vi "Generate INL Straight Lines.vi"(0 "Actual voltage array":dbl[](array[numeric]), 5 "INL Method":T1, 11 "Error In":errorcluster) -> (4 "Straight Line":dbl[](graph), 15 "Error Out":errorcluster)   [LabVIEW 2023]
doc: "The VI generates the best fit or end point straight line for INL calculation."
uses:
  Typedef/INL Method.ctl
  <vilib>/Analysis/NI_AALPro.lvlib
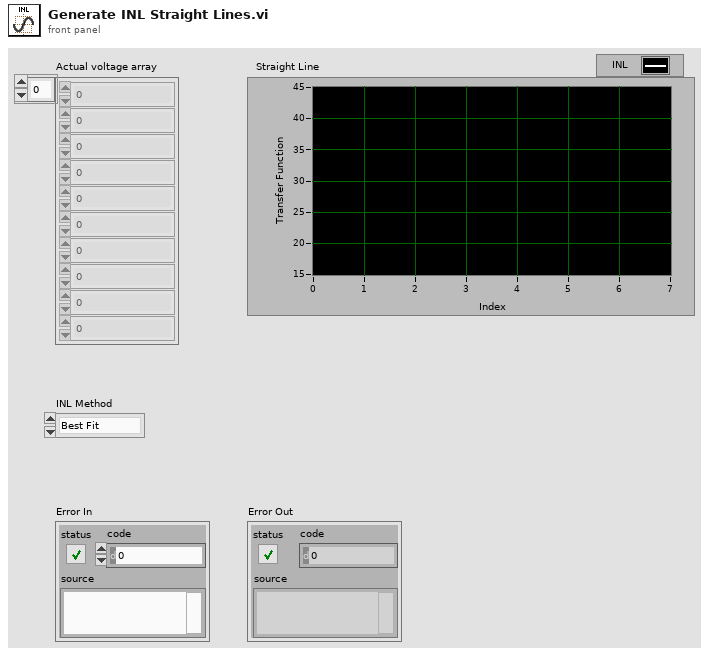
[diagram p1: front panel]
types:
  T1 = typedef "INL Method.ctl" = enum16{"Best Fit", "End Point"}
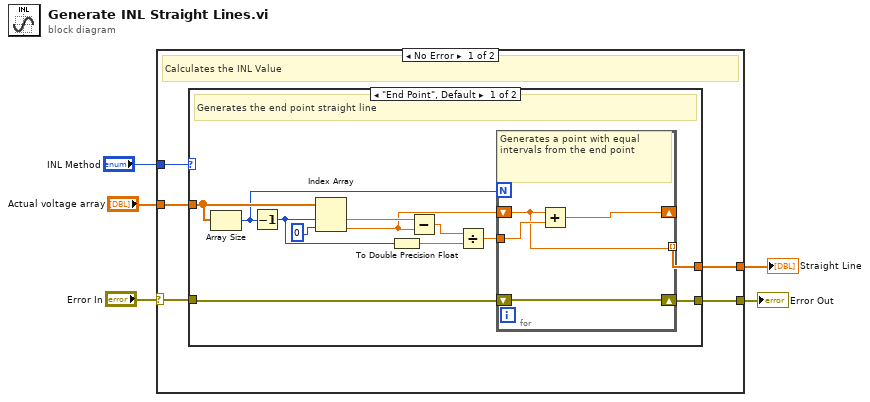
[diagram p0: block diagram]
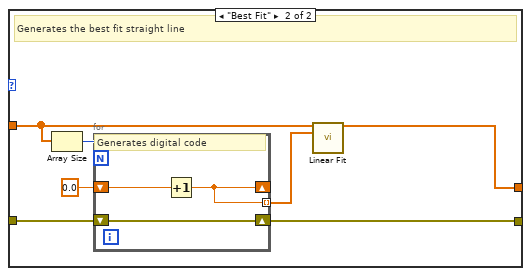
[diagram p2: hidden frame]
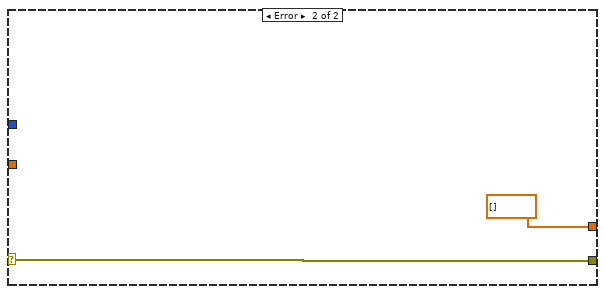
[diagram p3: hidden frame]
diagram:
  n1 = case shown="No Error" "Error In" {
    selector: "Error In" -> [w7 w38]
    tunnel: [w6 w38] -> w4
    tunnel: "Actual voltage array" -> [w10 _]
    tunnel: "INL Method" -> [w9 _]
    tunnel: [w8 dbl[] [] ("Best Linear Fit")] -> w1
    frame No Error {
      # "Calculates the INL Value"
      n2 = case shown="\"End Point\", Default" w9 {
        tunnel: [w15 w29] -> w8
        tunnel: w10 -> [w17 w32]
        tunnel: w7 -> [w12 w28]
        tunnel: [w11 w27] -> w6
        frame "End Point", Default {
          # "Generates the end point straight line"
          n3 = Array Size(array=w17) -> (size(s)=w13:i32)
          n4 = Decrement(x=w13) -> (x-1=w16:i32)
          n5 = Index Array(array=w17, index #1=w16, index #2=0 ("index")) -> (element #1=w20:dbl, element #2=w14:dbl)
          n6 = To Double Precision Float(number=w16) -> (double precision float=w18:dbl)
          n7 = Subtract(x=w20, y=w14) -> (x-y=w19:dbl)
          n8 = Divide(x=w19, y=w18) -> (x/y=w22:dbl)
          n9 = for {
            N: w13 -> [_]
            shift-right: [w25] -> _
            shift-left: w14 -> [w24]
            tunnel: w22 -> [w26]
            tunnel: [w24] -> w15 mode=indexing
            shift-right: [w23] -> w11
            shift-left: w12 -> [w23]
            # "Generates a point with equal intervals from the end point"
            n10 = Add(x=w24, y=w26) -> (x+y=w25:dbl)
          }
        }
        frame "Best Fit" {
          # "Generates the best fit straight line"
          n11 = Array Size(array=w32) -> (size(s)=w33:i32)
          n12 = for {
            N: w33 -> [_]
            shift-right: [w35] -> _
            shift-left: 0.0 -> [w36]
            tunnel: [w35] -> w30 mode=indexing
            shift-right: [w34] -> w27
            shift-left: w28 -> [w34]
            # "Generates digital code"
            n13 = Increment(x=w36) -> (x+1=w35:dbl)
          }
          n14 = call <vilib>:"Linear Fit.vi"("Y"=w32, "X"=w30) -> ("Best Linear Fit"=w29:dbl[])  [unwired: 9 in, 4 out]
        }
      }
    }
    frame Error {
    }
  }
  "Error Out" <- w4
  "Straight Line" <- w1
